vi "createTestCaseXMLReport_Helper.vi"(8 "error in (no error)":errorcluster, 10 "remaining elements (internal - do not use)":cluster{"Type":string, "Data":variant}[](array[cluster])) -> (0 "error out":errorcluster, 2 "XML string":string)   [LabVIEW 2013, in "_TextTestResult.JUnitXML.lvclass"]
uses:
  _TextTestResult.JUnitXML.lvclass
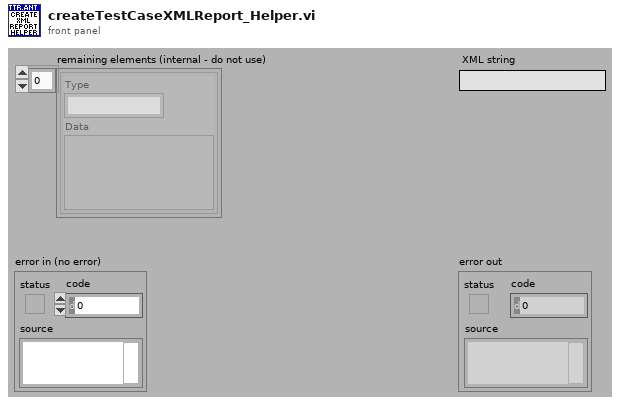
[diagram p1: front panel]
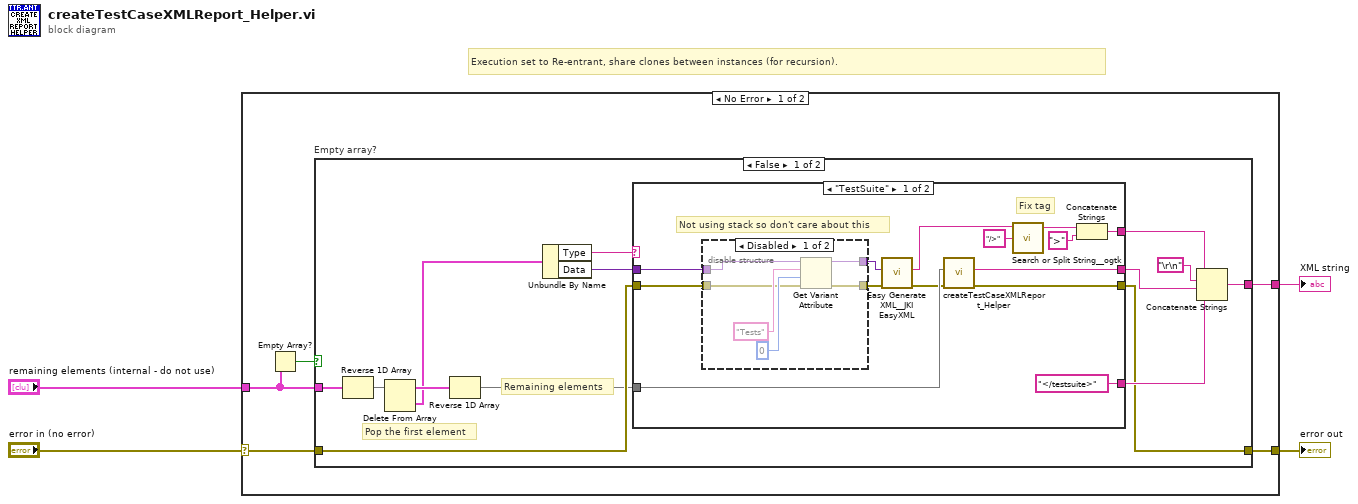
[diagram p0: block diagram]
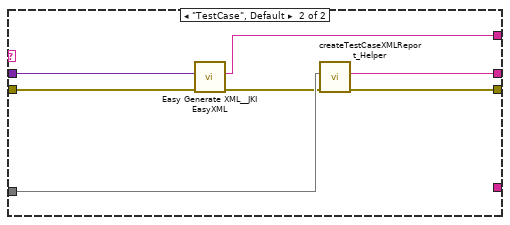
[diagram p3: hidden frame]
diagram:
  # "Execution set to Re-entrant, share clones between instances (for recursion)."
  n1 = case shown="No Error" "error in (no error)" {
    selector: "error in (no error)" -> [w9 w54]
    tunnel: [w5 w54] -> w3
    tunnel: "remaining elements (internal - do not use)" -> [w8 _]
    tunnel: [w6 _] -> w1
    frame No Error {
      n2 = Empty Array?(array=w8) -> (empty?=w7:bool)
      n3 = case "Empty array?" shown="False" w7 {
        tunnel: w9 -> [w21 w53]
        tunnel: w8 -> [w18 _]
        tunnel: [w13 _] -> w6
        tunnel: [w12 w53] -> w5
        frame False {
          # "Remaining elements"
          # "Pop the first element"
          n4 = Reverse 1D Array(array=w18) -> (reversed array=w17:cluster{"Type":string, "Data":variant}[])
          n5 = Delete From Array(array=w17) -> (deleted portion=w15:cluster{"Type":string, "Data":variant}, array with subset deleted=w16:cluster{"Type":string, "Data":variant}[])  [unwired: 2 in]
          n6 = Reverse 1D Array(array=w16) -> (reversed array=w14:cluster{"Type":string, "Data":variant}[])
          n7 = Unbundle By Name(w15) -> ("Type"=w23:string, "Data"=w22:variant)
          n8 = case shown="\"TestSuite\"" w23 {
            tunnel: w22 -> [w36 w52]
            tunnel: w21 -> [w35 w51]
            tunnel: [w33 w47] -> w20
            tunnel: ["</testsuite>" _] -> w19
            tunnel: w14 -> [w31 w50]
            tunnel: [w32 w48] -> w12
            tunnel: [w27 w46] -> w11
            frame "TestSuite" {
              # "Fix tag"
              # "Not using stack so don't care about this"
              n9 = disable-structure shown="Disabled" {
                disable-tunnel: w36 -> [w41 w44]
                disable-tunnel: w35 -> [w40 w45]
                disable-tunnel: [w39 w44] -> w34
                disable-tunnel: [w38 w45] -> w25
                frame Disabled {
                  n10 = Get Variant Attribute(Variant=w41, name="Tests", default value (empty Variant)=0 ("size(s)"), error in=w40) -> (duplicate Variant=w39:variant, error out=w38:errorcluster)  [unwired: 2 out]
                }
                frame Enabled {
                }
              }
              n11 = call <vilib>:"Easy Generate XML__JKI EasyXML.vi"("error in (no error)"=w25, "LabVIEW Data"=w34) -> ("error out"=w24:errorcluster, "XML String"=w26:string)  [unwired: 8 in]
              n12 = call "createTestCaseXMLReport_Helper.vi"("error in (no error)"=w24, "remaining elements (internal - do not use)"=w31) -> ("error out"=w32:errorcluster, "XML string"=w33:string)  [unwired: 8 in]
              n13 = call <userlib>:"Search or Split String__ogtk.vi"("search string/char (-)"="/>", "string"=w26) -> ("substring before match"=w29:string)  [unwired: 1 in, 2 out]
              n14 = Concatenate Strings(w29, ">" ("string")) -> (w27:string)
            }
            frame "TestCase", Default {
              n15 = call <vilib>:"Easy Generate XML__JKI EasyXML.vi"("error in (no error)"=w51, "LabVIEW Data"=w52) -> ("error out"=w49:errorcluster, "XML String"=w46:string)  [unwired: 8 in]
              n16 = call "createTestCaseXMLReport_Helper.vi"("error in (no error)"=w49, "remaining elements (internal - do not use)"=w50) -> ("error out"=w48:errorcluster, "XML string"=w47:string)  [unwired: 8 in]
            }
          }
          n17 = Concatenate Strings(w11, "\r\n", w20, w19) -> (w13:string)
        }
        frame True {
          # "Base case - finished."
        }
      }
    }
    frame Error {
    }
  }
  "error out" <- w3
  "XML string" <- w1
